vi "DAQ.vi"() -> ()   [LabVIEW 2013]
uses:
  <vilib>/DAQmx/read.llb/DAQmx Read (Analog 2D DBL NChan NSamp).vi
  <vilib>/DAQmx/create/channels.llb/DAQmx Create Channel (AI-Voltage-Basic).vi
  <vilib>/DAQmx/configure/timing.llb/DAQmx Timing (Sample Clock).vi
  <vilib>/DAQmx/configure/trigger.llb/DAQmx Start Trigger (Digital Edge).vi
  <vilib>/DAQmx/miscellaneous.llb/DAQmx Fill In Error Info.vi
panel:
  out "Last file written":path caption="Filename Out"
  in  "Filename":path=path "Cat_X/Cat_X.lvm"
  in  "Acquisition Time (s)":dbl
  in  "Channel 2":tag
  out "Waveform Graph":dbl[][](graph)
  in  "Trigger Source":tag
  in  "Sampling Rate (Hz)":dbl=1000.0 format="%0.2f"
  in  "Minimum value (V)":dbl=-5.0 format="%0.2f"
  in  "Maximum value (V)":dbl=5.0 format="%0.2f"
  in  "Channel 1":tag
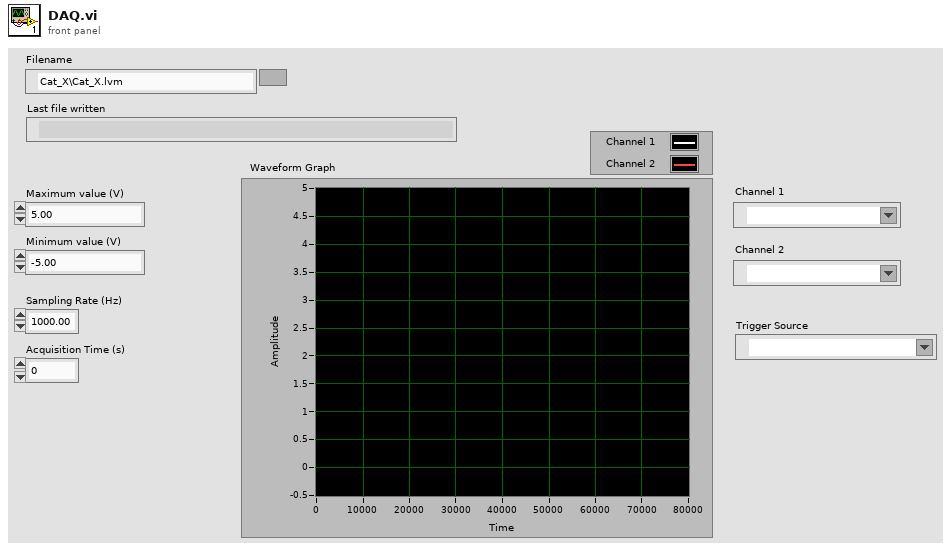
[diagram p1: front panel]
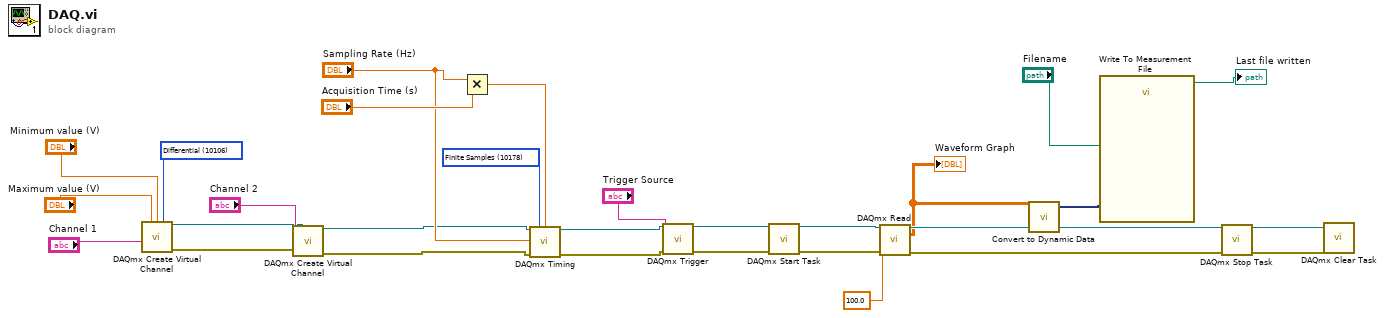
[diagram p0: block diagram]
diagram:
  w4 = 10106 items=["default"=-1, "RSE"=10083, "NRSE"=10078, "Differential"=10106, "Pseudodifferential"=12529] ("input terminal configuration")
  w16 = 10178 items=["Finite Samples"=10178, "Continuous Samples"=10123, "Hardware Timed Single Point"=12522] ("sample mode")
  n1 = call-poly <vilib>:"DAQmx Create Virtual Channel.vi"("maximum value"="Maximum value (V)", "minimum value"="Minimum value (V)", "input terminal configuration"=w4, "physical channels"="Channel 1") -> ("task out"=w18:refnum<k21>, "error out"=w17:errorcluster)  [unwired: 10 in]
  n2 = call-poly <vilib>:"DAQmx Create Virtual Channel.vi"("task in"=w18, "physical channels"="Channel 2", "error in"=w17) -> ("task out"=w3:refnum<k21>, "error out"=w2:errorcluster)  [unwired: 11 in]
  n3 = Multiply(x="Sampling Rate (Hz)", y="Acquisition Time (s)") -> (x*y=w8:dbl)
  n4 = call-poly <vilib>:"DAQmx Timing.vi"("task/channels in"=w3, "sample mode"=w16, "samples per channel"=w8, "rate"="Sampling Rate (Hz)", "error in"=w2) -> ("task out"=w13:refnum<k21>, "error out"=w12:errorcluster)  [unwired: 9 in]
  n5 = call-poly <vilib>:"DAQmx Trigger.vi"("task/channels in"=w13, "source"="Trigger Source", "error in"=w12) -> ("task out"=w11:refnum<k21>, "error out"=w10:errorcluster)  [unwired: 11 in]
  n6 = call <vilib>:"DAQmx Start Task.vi"("task/channels in"=w11, "error in"=w10) -> ("task out"=w24:refnum<k21>, "error out"=w25:errorcluster)  [unwired: 12 in]
  n7 = call-poly <vilib>:"DAQmx Read.vi"("task/channels in"=w24, "timeout"=100.0, "error in"=w25) -> ("task out"=w23:refnum<k21>, "data"=w15:dbl[][], "error out"=w22:errorcluster)  [unwired: 10 in]
  "Waveform Graph" <- w15
  n8 = call "Convert to Dynamic Data"("2D Array"=w15) -> ("Dynamic Data Type"=w14:dynamicdata)  [unwired: 3 in]
  n9 = call "Write To Measurement File"("Signals"=w14, "Filename"="Filename") -> ("Filename Out"=→"Last file written":path)  [unwired: 15 in, 2 out]
  n10 = call <vilib>:"DAQmx Stop Task.vi"("task/channels in"=w23, "error in"=w22) -> ("task out"=w21:refnum<k21>, "error out"=w20:errorcluster)  [unwired: 12 in]
  n11 = call <vilib>:"DAQmx Clear Task.vi"("task in"=w21, "error in"=w20) -> ()  [unwired: 13 in, 1 out]
